vi "- Test - Map VIMs.vi"() -> ()   [LabVIEW 2020]
uses:
  0236d640-7fb0-4049-b526-a4a0acec0d8d.vi
  14195457-9666-4654-9939-676a4b3105cd.vi
  081d8a99-1865-4d63-b336-dca8cbd81f72.vi
  158e93f0-6d83-44df-a97f-fd033c23c3c4.vi
  75fe9182-0039-4258-ba56-e63b77652130.vi
  081d8a99-1865-4d63-b336-dca8cbd81f72.vi/b0178052-0c48-4c9a-874f-40b592e34ac5.vi
  75fe9182-0039-4258-ba56-e63b77652130.vi/b0178052-0c48-4c9a-874f-40b592e34ac5.vi
panel:
  out "empty?":bool
  out "keys":string[](array[string])
  out "Keys":i32[](array[numeric])
  out "x = y?":bool
  out "map 2":map{i32, cluster{"bool":bool, "string":string}}(c390)
  out "map":T1(c390)
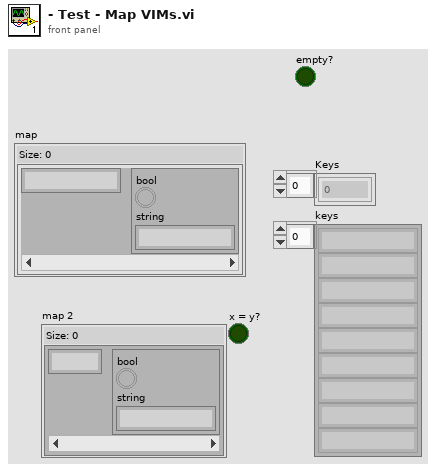
[diagram p1: front panel]
types:
  T1 = map{string, cluster{"bool":bool, "string":string}}
  T2 = cluster{"bool":bool, "string":string, "bool 2":bool, "Name":i32}
  T3 = cluster{"Name":string, "value":cluster{"bool":bool, "string":string}}[]
  T4 = map{string, cluster{"bool":bool, "string":string, "bool 2":bool, "Name":i32}}
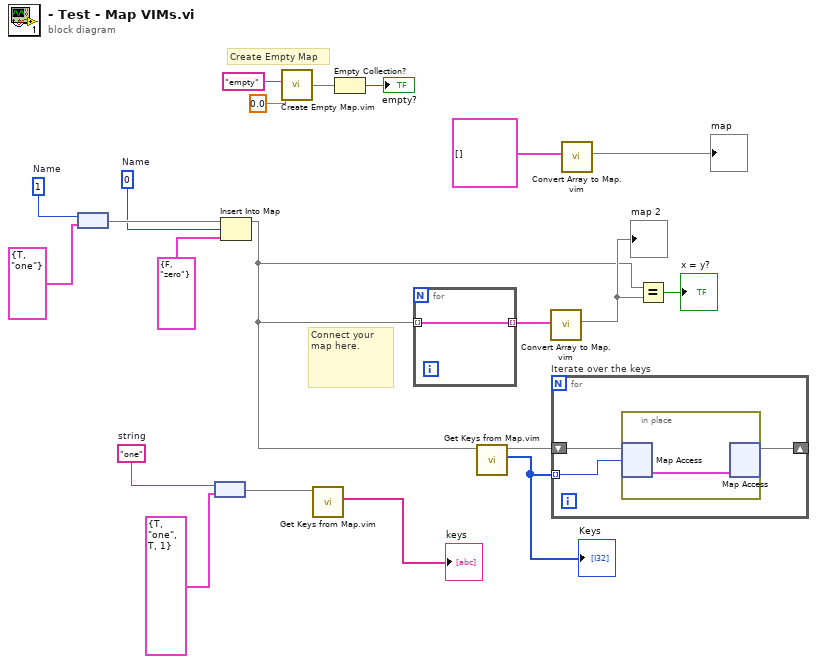
[diagram p0: block diagram]
diagram:
  w7 = "one"  # string
  w18 = 0  # Name
  w20 = 1  # Name
  # "Create Empty Map"
  # "Connect your map here."
  n1 = node(w20, cluster{"bool":bool, "string":string} {"bool"=TRUE, "string"="one"}) -> (w19:map{i32, cluster{"bool":bool, "string":string}})
  n2 = node(w7, T2 {"bool"=TRUE, "string"="one", "bool 2"=TRUE, "Name"=1}) -> (w6:T4)
  n3 = Insert Into Map(map in=w19, key=w18, value=cluster{"bool":bool, "string":string} {"bool"=FALSE, "string"="zero"}) -> (map out=w10:map{i32, cluster{"bool":bool, "string":string}})  [unwired: 2 out]
  n4 = call "Create Empty Map.vim"("value type"=0.0, "key type"="empty") -> ("empty map"=w2:map{string, dbl})  [unwired: 8 in]
  n5 = call "Get Keys from Map.vim"("map"=w6) -> ("keys"=→"keys":string[])  [unwired: 9 in, 1 out]
  n6 = Empty Collection?(1:w2) -> (0:→"empty?":bool)
  n7 = for {
    tunnel: [w22] -> w14 mode=indexing
    tunnel: w10 -> [w22] mode=indexing
  }
  n8 = call "Get Keys from Map.vim"("map"=w10) -> ("keys"=w11:i32[], "map out"=w9:map{i32, cluster{"bool":bool, "string":string}})  [unwired: 9 in]
  "Keys" <- w11
  n9 = call "Convert Array to Map.vim"("array"=w14) -> ("map"=w13:map{i32, cluster{"bool":bool, "string":string}})  [unwired: 10 in]
  "map 2" <- w13
  n10 = for "Iterate over the keys" {
    shift-right: [w23] -> _
    shift-left: w9 -> [w24]
    tunnel: w11 -> [w25] mode=indexing
    n11 = in-place {
      n12 = in-place-map #1(w24, w25) -> (w26:cluster{"bool":bool, "string":string})  [unwired: 1 in, 1 out]
      n13 = in-place-map #1(w26) -> (w23:map{i32, cluster{"bool":bool, "string":string}})  [unwired: 1 in, 2 out]
    }
  }
  n14 = call "Convert Array to Map.vim"("array"=T3 []) -> ("map"=→"map":T1)  [unwired: 10 in]
  n15 = Equal?(x=w10, y=w13) -> (x = y?=→"x = y?":bool)
